vi "unlock_semaphore.vi"(8 "error in (no error)":errorcluster, 11 "instrument in":refnum<class "instrument.lvclass">) -> (0 "error out":errorcluster, 3 "instrument out":refnum<class "instrument.lvclass">)   [LabVIEW 2017, in "instrument.lvclass"]
doc: "Uses a semaphore (private property of the instrument class) to restrict the communication to the instrument to one process at the time. This VI \"unlocks\" or releases the process/semaphore."
uses:
  instrument.lvclass
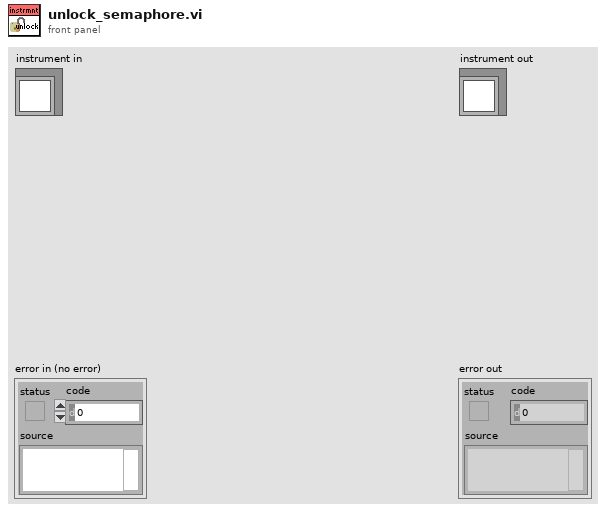
[diagram p1: front panel]
types:
  T1 = typedef "Semaphore RefNum" = refnum<k1>
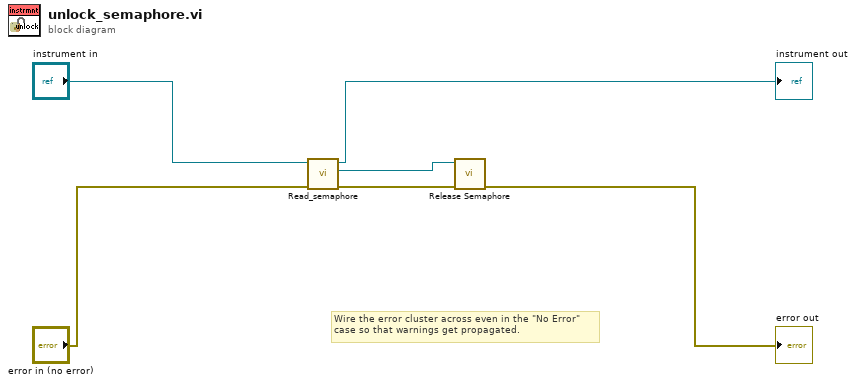
[diagram p0: block diagram]
diagram:
  # "Wire the error cluster across even in the \"No Error\"\ncase so that warnings get propagated."
  n1 = call-dynamic "Read_semaphore.vi"("error in (no error)"="error in (no error)", "instrument in"="instrument in") -> ("error out"=w1:errorcluster, "semaphore"=w2:T1, "instrument out"=→"instrument out":refnum<class "instrument.lvclass">)  [unwired: 7 in]
  n2 = call <vilib>:"Release Semaphore.vi"("error in (no error)"=w1, "semaphore"=w2) -> ("error out"=→"error out":errorcluster)  [unwired: 4 in, 1 out]
